vi "poly_asynch_wait_wait.vi"(6 "check interval (50 ms)":u32=50, 7 "restart asynch wait? (F)":bool, 8 "error in":errorcluster, 9 "timeout":i32, 10 "asynch wait ref in":T1) -> (0 "error out":errorcluster, 1 "timed out?":bool, 2 "asynch wait ref out":T1)   [LabVIEW 2015]
uses:
  cores/asynch_wait_ref.ctl
  cores/boolean_notifier.ctl
  poly_timing_tools_eco_plus.vi
  poly_loop_timeout_bool.vi
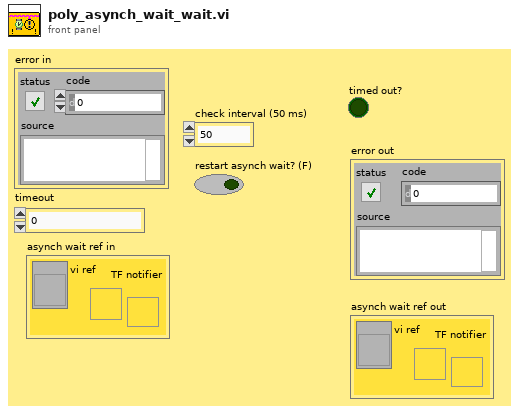
[diagram p1: front panel]
types:
  T1 = typedef "asynch_wait_ref.ctl" = cluster{"vi ref":refnum<vi>, "TF notifier":T2}
  T2 = typedef "boolean_notifier.ctl" = refnum<notifier>
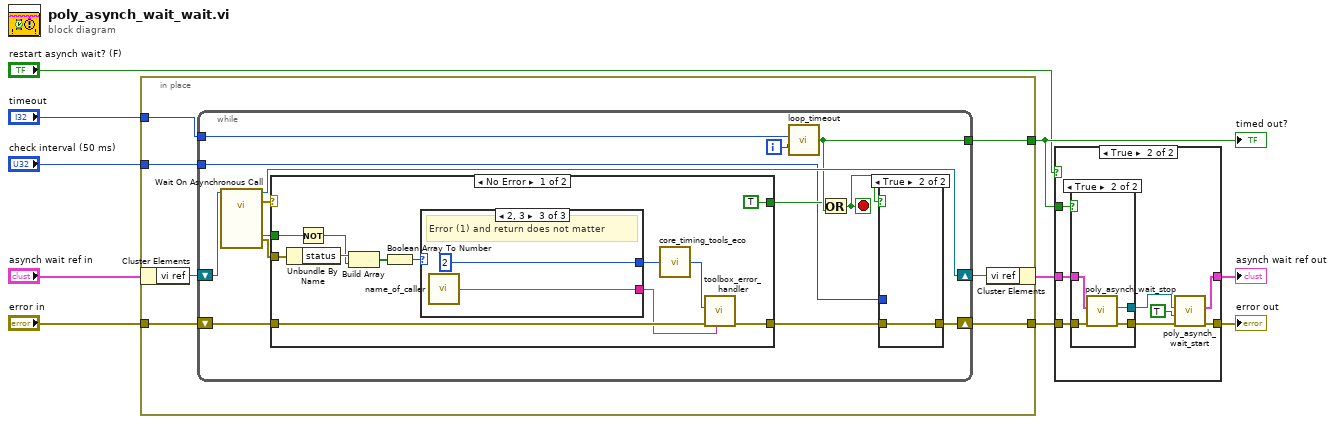
[diagram p0: block diagram]
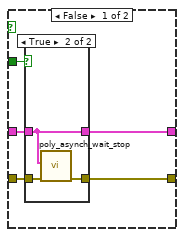
[diagram p2: hidden frame]
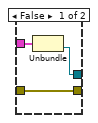
[diagram p4: hidden frame]
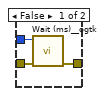
[diagram p5: hidden frame]
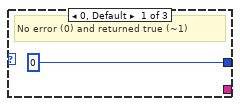
[diagram p6: hidden frame]
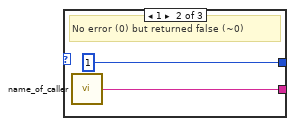
[diagram p7: hidden frame]
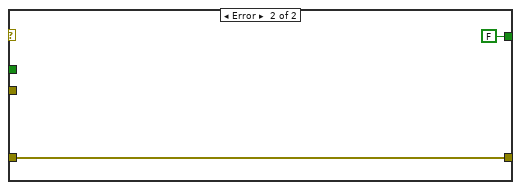
[diagram p8: hidden frame]
diagram:
  n1 = in-place {
    in-place-border: "timeout" -> [w16]
    in-place-border: [w15] -> w4
    in-place-border: "check interval (50 ms)" -> [w13]
    in-place-border: [w12] -> w2
    in-place-border: "error in" -> [w11]
    n2 = in-place-cluster #1("asynch wait ref in") -> ("vi ref"=w17:refnum<vi>)
    n3 = while {
      tunnel: w16 -> [w25]
      tunnel: [w23] -> w15
      shift-right: [w28] -> w14
      shift-left: w17 -> [w31]
      tunnel: w13 -> [w19]
      shift-right: [w20] -> w12
      shift-left: w11 -> [w26]
      i -> [w24]
      stop <- w18 stop-if-true
      n4 = call-by-ref "Wait On Asynchronous Call"(reference=w31) -> (reference out=w28:refnum<vi>, error out=w30:errorcluster, "Error out"=w29:errorcluster, "notification"=w27:bool)  [unwired: 9 in, 2 out]
      n5 = case shown="No Error" w30 {
        tunnel: w29 -> [w45 _]
        tunnel: [TRUE FALSE] -> w22
        tunnel: w27 -> [w41 _]
        tunnel: [w39 w53] -> w21
        tunnel: w26 -> [w46 w53]
        frame No Error {
          n6 = Unbundle By Name(w45) -> ("status"=w44:bool)
          n7 = Not(x=w41) -> (.not. x?=w40:bool)
          n8 = Build Array(w44, w40) -> (w43:bool[])
          n9 = Boolean Array To Number(Boolean array=w43) -> (number=w42:u32)
          n10 = case shown="2, 3" w42 {
            tunnel: [0 1 2] -> w38
            tunnel: [_ w49 w51] -> w36
            frame 0, Default {
              # "No error (0) and returned true (~1)"
            }
            frame 1 {
              # "No error (0) but returned false (~0)"
              n11 = call "name_of_caller.vi"() -> ("name of caller out"=w49:string)  [unwired: 4 in]
            }
            frame 2, 3 {
              # "Error (1) and return does not matter"
              n12 = call "name_of_caller.vi"() -> ("name of caller out"=w51:string)  [unwired: 4 in]
            }
          }
          n13 = call-poly "core_timing_tools_eco.vi"("code (w/out eco)"=w38) -> ("code (+ eco)"=w37:i32)  [unwired: 4 in]
          n14 = call "toolbox_error_handler.vi"("name of caller in (you)"=w36, "error in (no error)"=w46, "code (0 = no error)"=w37) -> ("error out"=w39:errorcluster)  [unwired: 7 in, 1 out]
        }
        frame Error {
        }
      }
      n15 = call-poly "loop_timeout.vi"("timeout (2k ms)"=w25, "i (reset @ 0)"=w24) -> ("timeout"=w23:bool)  [unwired: 5 in]
      n16 = Or(x=w22, y=w23) -> (x .or. y?=w18:bool)
      n17 = case shown="True" w18 {
        tunnel: w21 -> [w34 w35]
        tunnel: [w33 w35] -> w20
        tunnel: w19 -> [w32 _]
        frame False {
          n18 = call <userlib>:"Wait (ms)__ogtk.vi"("error in (no error)"=w34, "milliseconds to wait"=w32) -> ("error out"=w33:errorcluster)  [unwired: 8 in, 1 out]
        }
        frame True {
        }
      }
    }
    n19 = in-place-cluster #1("vi ref"=w14) -> (w7:T1)
  }
  "timed out?" <- w4
  n20 = case shown="True" "restart asynch wait? (F)" {
    tunnel: w7 -> [w57 w69]
    tunnel: [w56 w68] -> w6
    tunnel: w2 -> [w59 w67]
    tunnel: [w58 w66] -> w5
    tunnel: w4 -> [w55 w65]
    frame False {
      n21 = case shown="True" w55 {
        tunnel: w57 -> [w60 w62]
        tunnel: w59 -> [w61 w64]
        tunnel: [w61 w63] -> w58
        tunnel: [w60 w62] -> w56
        frame False {
        }
        frame True {
          n22 = call "poly_asynch_wait_stop.vi"("error in"=w64, "asynch wait ref in"=w62) -> ("error out"=w63:errorcluster)  [unwired: 8 in, 1 out]
        }
      }
    }
    frame True {
      n23 = case shown="True" w65 {
        tunnel: [w73 w79] -> w71
        tunnel: [w74 w78] -> w70
        tunnel: w69 -> [w75 w77]
        tunnel: w67 -> [w73 w76]
        frame False {
          n24 = Unbundle(w75) -> ("TF notifier"=w74:T2)  [unwired: 1 out]
        }
        frame True {
          n25 = call "poly_asynch_wait_stop.vi"("error in"=w76, "asynch wait ref in"=w77) -> ("error out"=w79:errorcluster, "notifier"=w78:T2)  [unwired: 8 in]
        }
      }
      n26 = call "poly_asynch_wait_start.vi"("error in"=w71, "ignore previous (T)"=TRUE, "notifier (create)"=w70) -> ("error out"=w66:errorcluster, "asynch wait ref out"=w68:T1)  [unwired: 5 in, 2 out]
    }
  }
  "asynch wait ref out" <- w6
  "error out" <- w5
